vi "FileLockAlert.vi"(0 "Retry Cycle Count":i32) -> ()   [LabVIEW 2021]
panel:
  # "File conflict ALERT"
  # "The archive file is locked\nby another user. This error\nshould resolve itself. If you\nare still seeing this error \nwindow after 100 cycles \ncontact IT team."
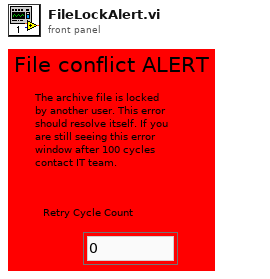
[diagram p1: front panel]
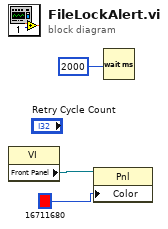
[diagram p0: block diagram]
diagram:
  n1 = property class="VI"() -> ("Front Panel"=w3:refnum<vi>)  [unwired: 2 in, 2 out]
  n2 = property class="Pnl"(reference=w3, "Color"=u32 16711680) -> ()  [unwired: 1 in, 2 out]
  n3 = Wait (ms)(milliseconds to wait=2000) -> ()  [unwired: 1 out]
